vi "HeartRate_Global.vi"() -> ()   [LabVIEW 2015]
panel:
  in  "got rate?":bool
  in  "rate":dbl
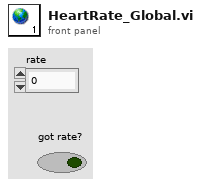
[diagram p1: front panel]
diagram:
